vi "ERR Initialize.vi"(11 "Error In (no error)":errorcluster) -> (8 "Error Description File":string, 15 "Error Out":errorcluster)   [LabVIEW 2011]
doc: "This VIs purpose is the initialization of error handling. It reads the error description file and loads a global with: error codes, error descriptions, and error levels. It also clears the \"last error\" global entry.\n\nThe input requirements are from the \"USRinit.vi\" and all paths are checked there.\n\nThe format of the error description file is as follows:\n\n[<error code>,\\t<error level>,\\t<error description>\\r]\n\nThis vi was created by David Gianetto, contact me with any problems, questions, etc."
uses:
  File IO/Type Defs/FILE Type Enum.ctl
  Globals/ERR Error Global.vi
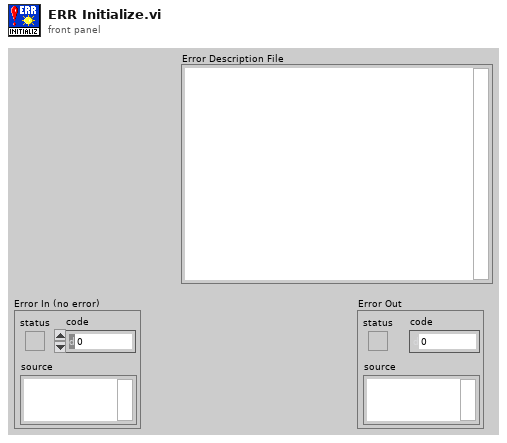
[diagram p1: front panel]
types:
  T1 = typedef "FILE Type Enum.ctl" = enum16{"Text", "Spreadsheet"}
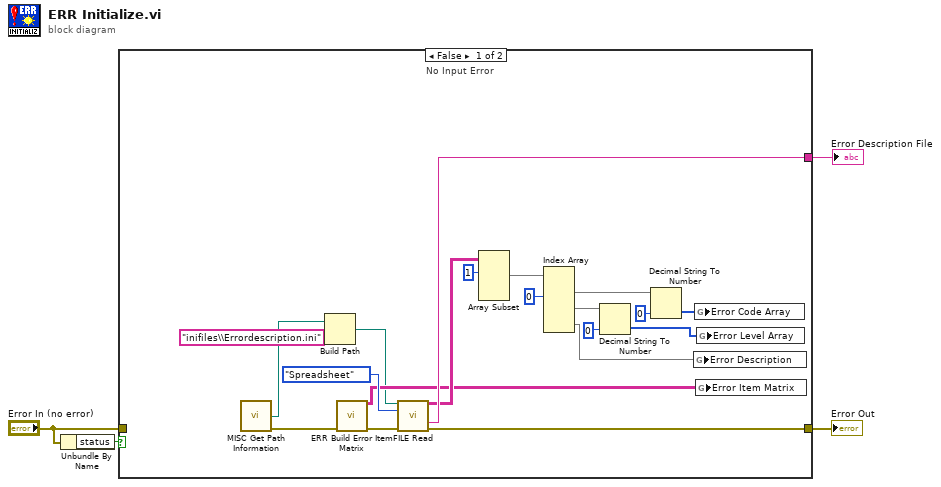
[diagram p0: block diagram]
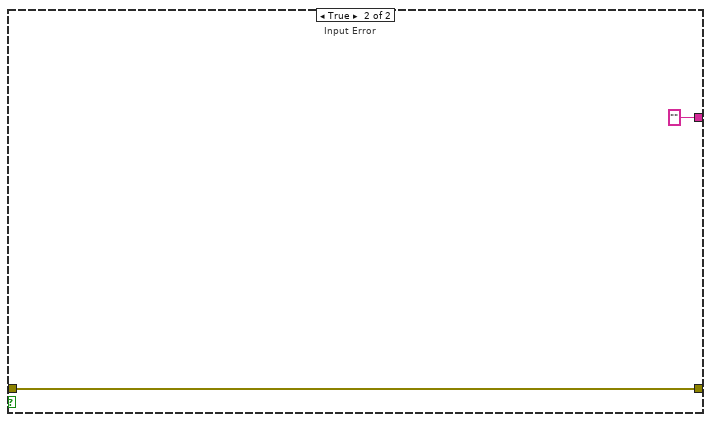
[diagram p2: hidden frame]
diagram:
  n1 = Unbundle By Name("Error In (no error)") -> ("status"=w4:bool)
  n2 = case shown="False" w4 {
    tunnel: "Error In (no error)" -> [_ w26]
    tunnel: [w24 w26] -> w3
    tunnel: [w22 "" ("Output String")] -> w2
    frame False {
      # "No Input Error"
      n3 = call "MISC Get Path Information.vi"() -> ("Support Directory"=w9:path, "Error Out"=w6:errorcluster)  [unwired: 1 in, 13 out]
      n4 = Build Path(base path=w9, name or relative path="inifiles\\Errordescription.ini") -> (appended path=w8:path)
      n5 = call "ERR Build Error Item Matrix.vi"("Error In (No Error)"=w6) -> ("Error Item Matrix"=w10:string[][], "Error Out"=w5:errorcluster)  [unwired: 1 in, 12 out]
      n6 = call "FILE Read.vi"("File Path (dialog if empty)"=w8, "File Type (text)"=FILE_Type_Enum."Spreadsheet", "Error In (no error)"=w5) -> ("Spreadsheet Data (all)"=w14:string[][], "Output String"=w22:string, "Error Out"=w24:errorcluster)  [unwired: 4 in, 6 out]
      n7 = Array Subset(array=w14, index (row)=1) -> (w20:string[][])  [unwired: 3 in]
      n8 = Index Array(array=w20, index (col) #1=0 ("Disabled Index (col)")) -> (element #1=w18:string[], element #2=w17:string[], element #3=w11:string[])  [unwired: 5 in]
      n9 = Decimal String To Number(string=w17, default (0L)=0 ("Disabled Index (col)")) -> (number=w12:i32[])  [unwired: 2 out]
      n10 = Decimal String To Number(string=w18, default (0L)=0 ("Disabled Index (col)")) -> (number=w13:i32[])  [unwired: 2 out]
      n11 = global write "ERR Error Global.vi" "Error Description"(w11) -> ()
      n12 = global write "ERR Error Global.vi" "Error Code Array"(w13) -> ()
      n13 = global write "ERR Error Global.vi" "Error Item Matrix"(w10) -> ()
      n14 = global write "ERR Error Global.vi" "Error Level Array"(w12) -> ()
    }
    frame True {
      # "Input Error"
    }
  }
  "Error Out" <- w3
  "Error Description File" <- w2
